vi "config opr.vi"(4 "name or relative path":string="config\\chconfig.cfg", 5 "key":string="default config\\ChConfig.cfg", 6 "Not project Path?":bool, 7 "project path":path, 8 "error in":errorcluster, 9 "Chanel":T1 {"CHS"."display" format="%b"}, 10 "defaultPath":path, 11 "config opr":T4) -> (0 "error out":errorcluster, 2 "chconfig data":T1 {"CHS"."display" format="%b"})   [LabVIEW 2011]
uses:
  config opr.ctl
  contable.ctl
  CHS.ctl
  singlechtype.ctl
  <vilib>/Utility/file.llb/Read From Spreadsheet File (string).vi
panel:
  in  "Enum":enum16{"cfg", "excel"}(ring)=enum."excel"
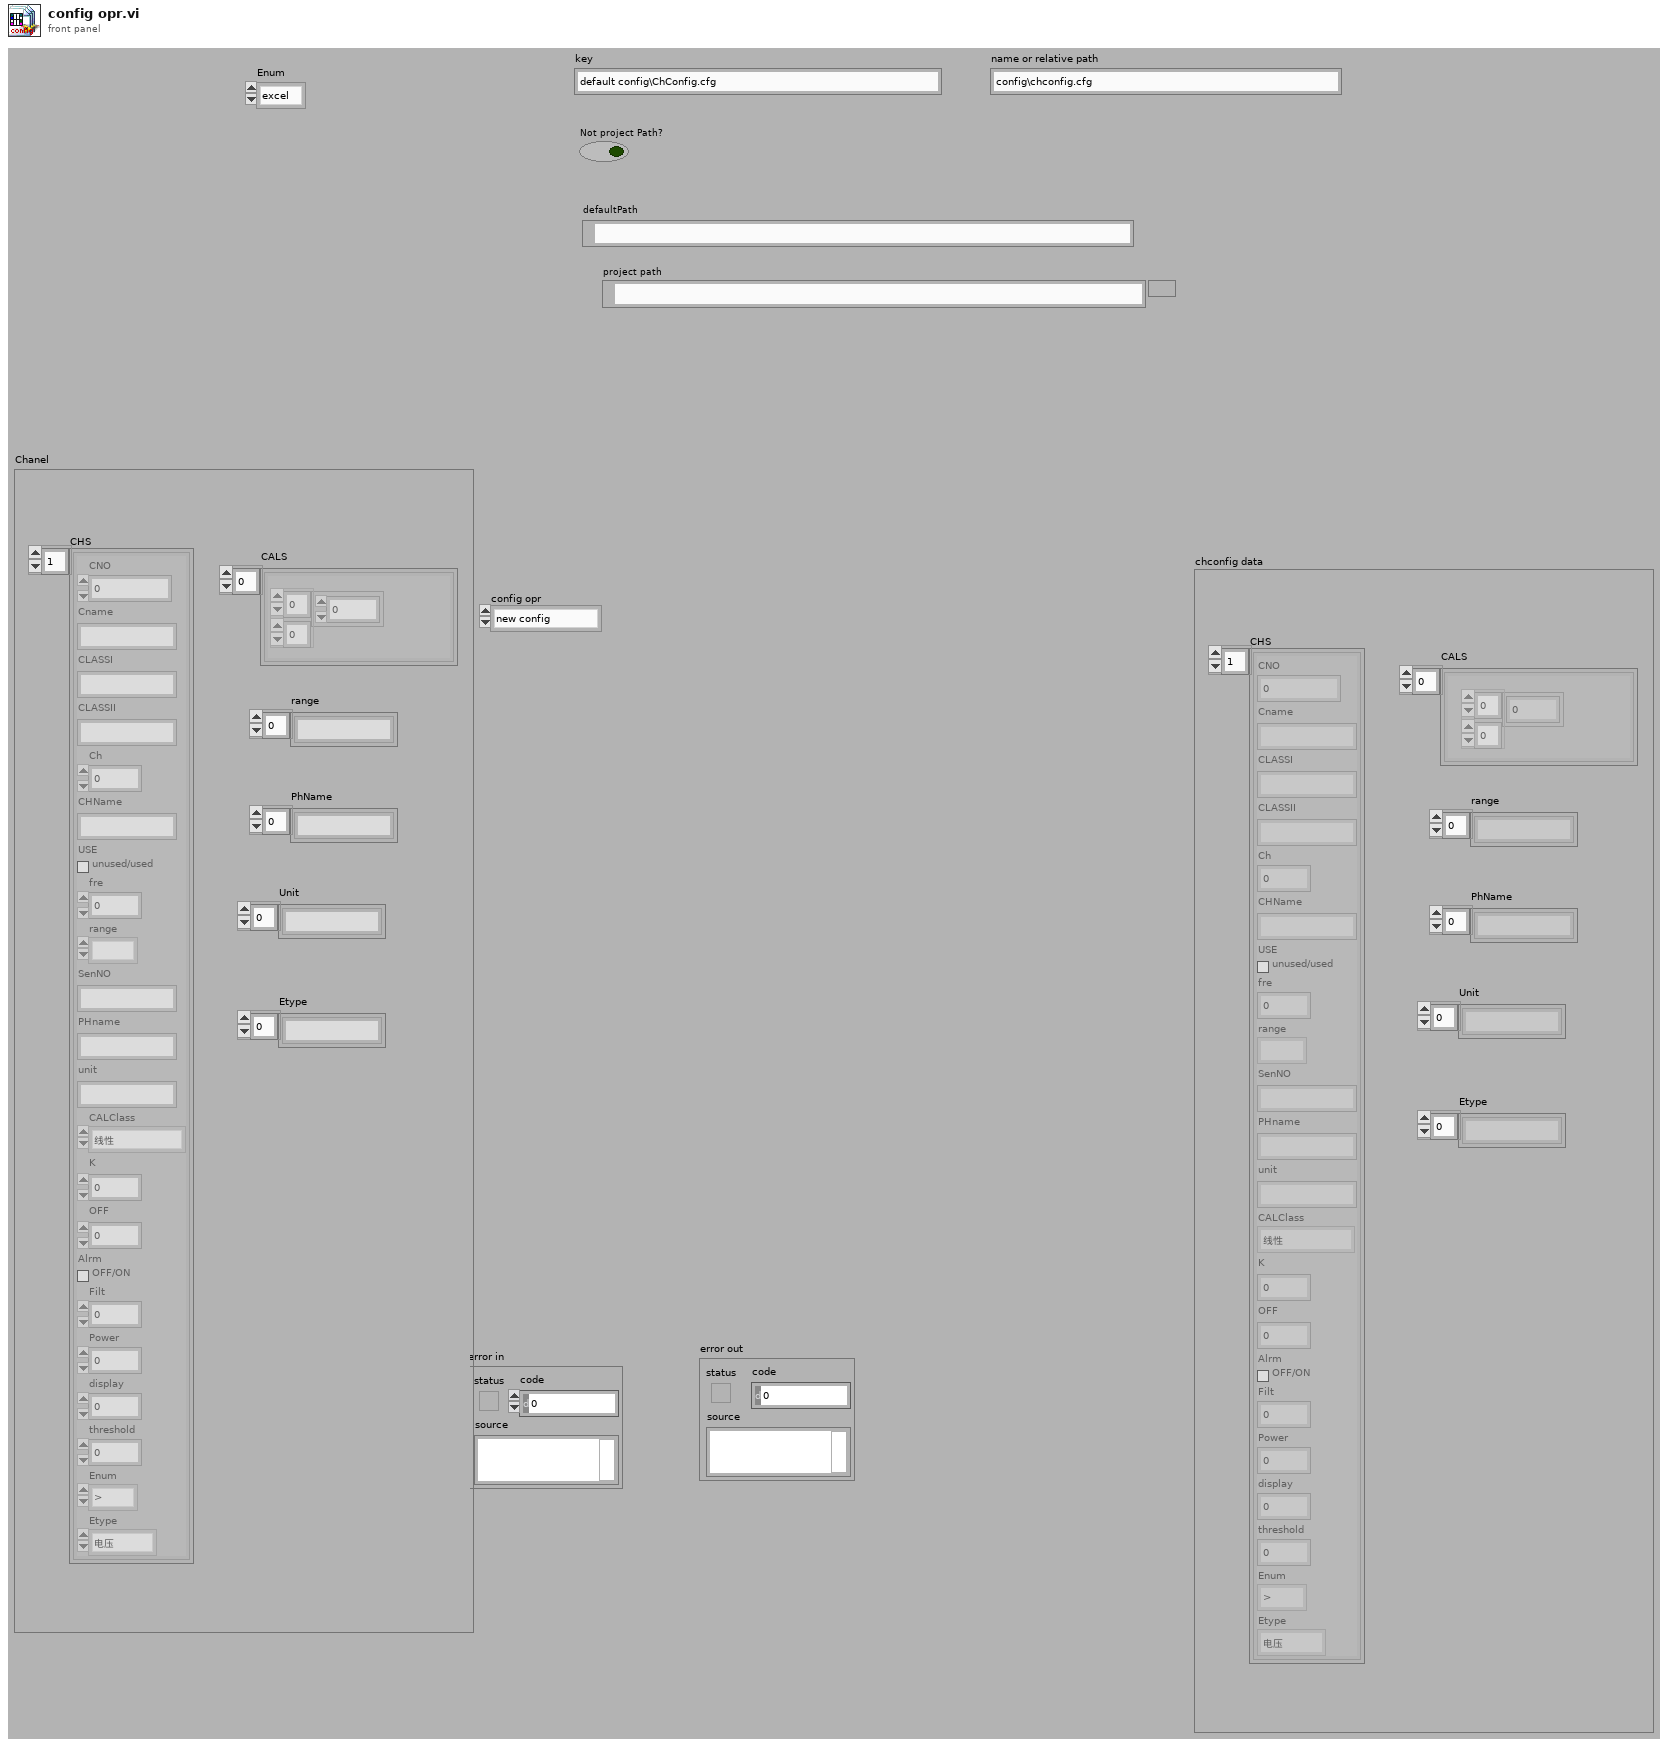
[diagram p1: front panel]
types:
  T1 = typedef "contable.ctl" = cluster{"CHS":T2, "CALS":cluster{"Array":dbl[][]}[], "range":string[], "PhName":string[], "Unit":string[], "Etype":string[]}
  T2 = typedef "CHS.ctl" = T3[]
  T3 = typedef "singlechtype.ctl" = cluster{"CNO":u8, "Cname":string, "CLASSI":string, "CLASSII":string, "Ch":u8, "CHName":string, "USE":bool, "fre":dbl, "range":enum16{""}, "SenNO":string, "PHname":string, "unit":string, "CALClass":enum8{"线性", "查表", "公式"}, "K":dbl, "OFF":dbl, "Alrm":bool, "Filt":dbl, "Power":u8, "display":u8, "threshold ":dbl, "Enum":enum16{">", ">=", "<", "<=", "<>(在范围内）", "><（在范围外）"}, "Etype":enum16{"电压", "电流", "电阻", "热电偶K", "热电偶T"}}
  T4 = typedef "config opr.ctl" = enum16{"new config", "read config", "write config", "close config", "write defaultconfig", ""}
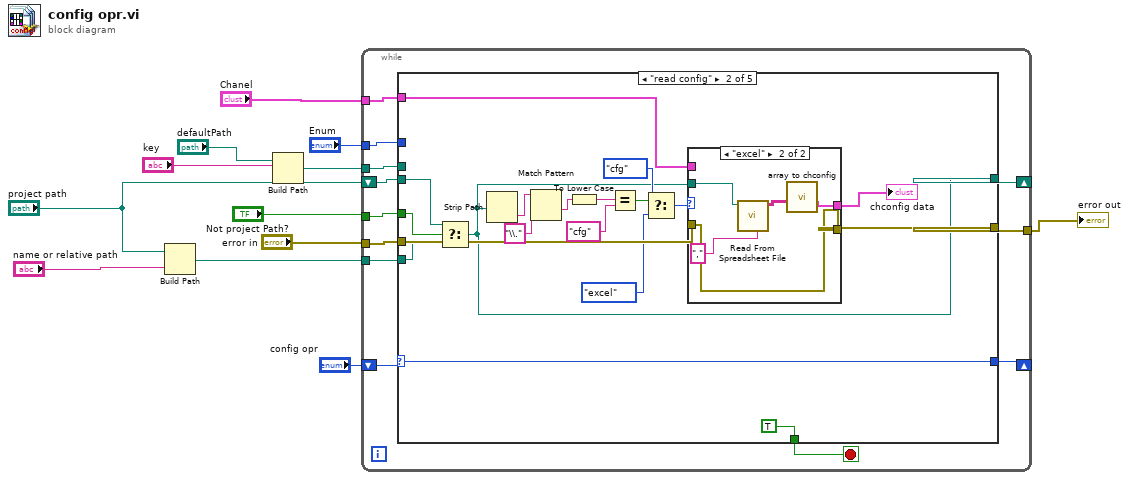
[diagram p0: block diagram]
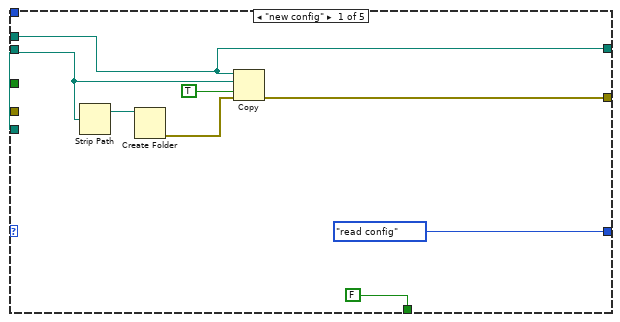
[diagram p2: hidden frame]
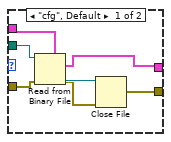
[diagram p3: hidden frame]
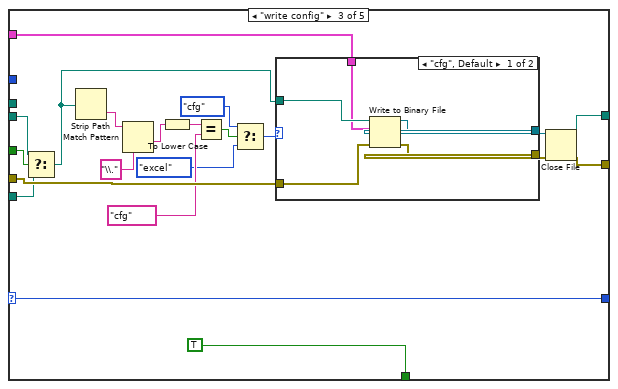
[diagram p4: hidden frame]
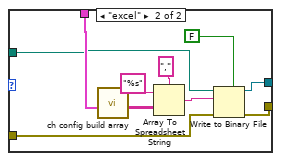
[diagram p5: hidden frame]
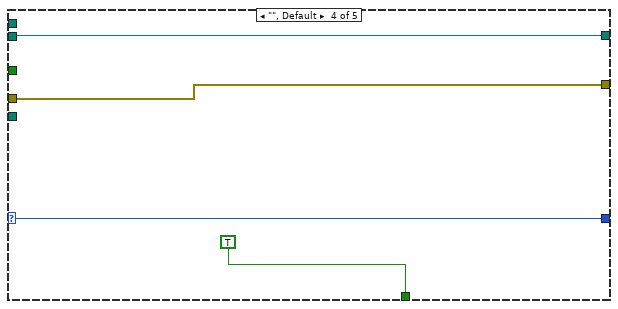
[diagram p6: hidden frame]
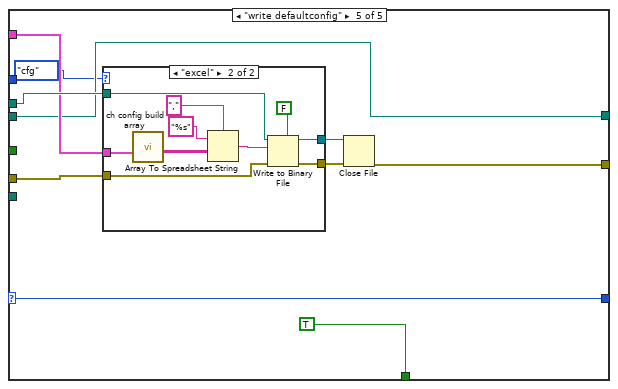
[diagram p7: hidden frame]
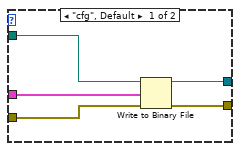
[diagram p8: hidden frame]
diagram:
  n1 = Build Path(base path="project path", name or relative path="name or relative path") -> (appended path=w6:path)
  n2 = Build Path(base path="defaultPath", name or relative path="key") -> (appended path=w11:path)
  n3 = while {
    tunnel: w11 -> [w24]
    tunnel: w6 -> [w23]
    tunnel: "error in" -> [w22]
    tunnel: [w20] -> w8
    shift-right: [w17] -> _
    shift-left: "project path" -> [w19]
    tunnel: "Chanel" -> [w18]
    shift-right: [w16] -> _
    shift-left: "config opr" -> [w21]
    tunnel: "Not project Path?" -> [w14]
    tunnel: "Enum" -> [w13]
    stop <- w15 stop-if-true
    n4 = case shown="\"read config\"" w21 {
      selector: w21 -> [_ w48 w79 w101 w106]
      tunnel: w24 -> [w26 _ _ _ w113]
      tunnel: w23 -> [w25 w45 w76 _ _]
      tunnel: w22 -> [_ w51 w84 w103 w109]
      tunnel: [w30 w43 w81 w103 w110] -> w20
      tunnel: w19 -> [_ w46 w77 w102 w107]
      tunnel: w18 -> [_ w50 w74 _ w108]
      tunnel: [w26 w36 w80 w102 w107] -> w17
      tunnel: [config_opr."read config" ("config opr") w48 w79 w101 w106] -> w16
      tunnel: [FALSE TRUE TRUE TRUE TRUE] -> w15
      tunnel: w14 -> [_ w44 w75 _ _]
      tunnel: w13 -> [_ _ _ _ _]
      frame "new config" {
        n5 = Strip Path(path=w25) -> (stripped path=w27:path)  [unwired: 1 out]
        n6 = Create Folder(path (use dialog)=w27) -> (error out=w31:errorcluster)  [unwired: 1 in, 3 out]
        n7 = Copy(8:w31, 9:TRUE ("overwrite (F)"), 10:w25, 11:w26) -> (0:w30:errorcluster)  [unwired: 3 out]
      }
      frame "read config" {
        n8 = Select(t=w46, s=w44, f=w45) -> (s? t:f=w36:path)
        n9 = Strip Path(path=w36) -> (name=w42:string)  [unwired: 1 out]
        n10 = Match Pattern(string=w42, regular expression="\\.") -> (after substring=w34:string)  [unwired: 4 out]
        n11 = To Lower Case(string=w34) -> (all lower case string=w39:string)
        n12 = Equal?(x=w39, y="cfg") -> (x = y?=w38:bool)
        n13 = Select(t=enum16{"cfg", "excel"}."cfg" ("Enum"), s=w38, f=enum16{"cfg", "excel"}."excel" ("Enum")) -> (s? t:f=w35:enum16{"cfg", "excel"})
        n14 = case shown="\"excel\"" w35 {
          tunnel: w51 -> [w58 w62]
          tunnel: w50 -> [w57 _]
          tunnel: [w56 w60] -> w49
          tunnel: w36 -> [w55 w63]
          tunnel: [w52 w62] -> w43
          frame "cfg", Default {
            n15 = Read from Binary File(5:w57, 8:w58, 11:w55) -> (0:w53:errorcluster, 2:w56:T1, 3:w54:refnum<file>)  [unwired: 1 in, 3 out]
            n16 = Close File(refnum=w54, error in=w53) -> (error out=w52:errorcluster)  [unwired: 1 out]
          }
          frame "excel" {
            n17 = call-poly <vilib>:"Read From Spreadsheet File.vi"("delimiter (\\t)"="," ("delimiter (Tab)"), "file path (dialog if empty)"=w63) -> ("all rows"=w61:string[][])  [unwired: 3 in, 6 out]
            n18 = call "array to chconfig.vi"("output array"=w61) -> ("configtable"=w60:T1)  [unwired: 10 out]
          }
        }
        "chconfig data" <- w49
      }
      frame "write config" {
        n19 = Select(t=w77, s=w75, f=w76) -> (s? t:f=w73:path)
        n20 = Strip Path(path=w73) -> (name=w72:string)  [unwired: 1 out]
        n21 = Match Pattern(string=w72, regular expression="\\.") -> (after substring=w64:string)  [unwired: 4 out]
        n22 = To Lower Case(string=w64) -> (all lower case string=w69:string)
        n23 = Equal?(x=w69, y="cfg") -> (x = y?=w68:bool)
        n24 = Select(t=enum16{"cfg", "excel"}."cfg" ("Enum"), s=w68, f=enum16{"cfg", "excel"}."excel" ("Enum")) -> (s? t:f=w65:enum16{"cfg", "excel"})
        n25 = case shown="\"cfg\", Default" w65 {
          tunnel: w84 -> [w89 w96]
          tunnel: [w88 w98] -> w83
          tunnel: [w87 w97] -> w82
          tunnel: w73 -> [w86 w90]
          tunnel: w74 -> [w85 w99]
          frame "cfg", Default {
            n26 = Write to Binary File(file (use dialog)=w86, data=w85, error in=w89) -> (refnum out=w88:refnum<file>, error out=w87:errorcluster)  [unwired: 2 in, 2 out]
          }
          frame "excel" {
            n27 = call "ch config build array.vi"("configtable"=w99) -> ("output array"=w94:string[][])  [unwired: 10 out]
            n28 = Array To Spreadsheet String(delimiter (Tab)=",", array=w94, 3:"%s" ("format string")) -> (spreadsheet string=w95:string)
            n29 = Write to Binary File(file (use dialog)=w90, data=w95, error in=w96, 5:FALSE ("prepend array or string size? (T)")) -> (refnum out=w98:refnum<file>, error out=w97:errorcluster)  [unwired: 2 in, 1 out]
          }
        }
        n30 = Close File(refnum=w83, error in=w82) -> (path=w80:path, error out=w81:errorcluster)
      }
      frame "", Default {
      }
      frame "write defaultconfig" {
        n31 = case shown="\"excel\"" enum16{"cfg", "excel"}."cfg" ("Enum") {
          tunnel: w113 -> [w118 w120]
          tunnel: [w117 w126] -> w112
          tunnel: [w116 w127] -> w111
          tunnel: w109 -> [w115 w128]
          tunnel: w108 -> [w114 w122]
          frame "cfg", Default {
            n32 = Write to Binary File(file (use dialog)=w118, data=w114, error in=w115) -> (refnum out=w117:refnum<file>, error out=w116:errorcluster)  [unwired: 4 out]
          }
          frame "excel" {
            n33 = call "ch config build array.vi"("configtable"=w122) -> ("output array"=w125:string[][])  [unwired: 10 out]
            n34 = Array To Spreadsheet String(delimiter (Tab)=",", array=w125, 3:"%s" ("format string")) -> (spreadsheet string=w121:string)
            n35 = Write to Binary File(file (use dialog)=w120, data=w121, error in=w128, 5:FALSE ("prepend array or string size? (T)")) -> (refnum out=w126:refnum<file>, error out=w127:errorcluster)  [unwired: 3 out]
          }
        }
        n36 = Close File(refnum=w112, error in=w111) -> (error out=w110:errorcluster)  [unwired: 1 out]
      }
    }
  }
  "error out" <- w8
